vi "Create False Constant.vi"(5 "Sink":refnum<vi>, 6 "relative position/next to refnum":T1, 8 "error in (no error)":errorcluster, 11 "Diagram":refnum<vi>) -> (0 "error out":errorcluster, 2 "Output Terminal":refnum<vi>, 3 "Constant ref":refnum<vi>)   [LabVIEW 2012, in "Scripting Tools.lvlib"]
uses:
  Scripting Tools.lvlib
  <vilib>/Utility/miscctls.llb/LVPointTypeDef.ctl
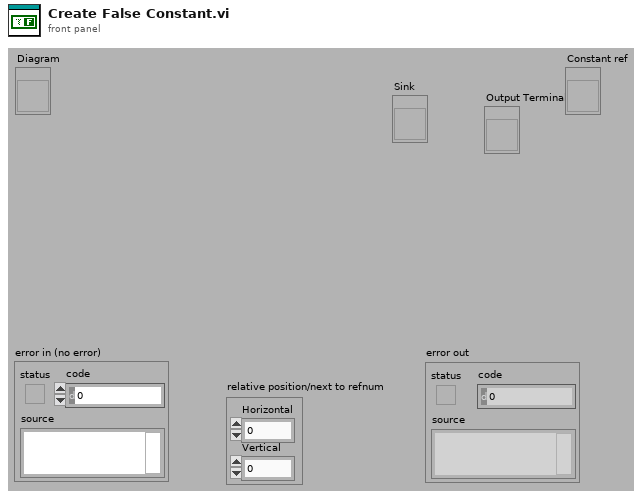
[diagram p1: front panel]
types:
  T1 = typedef "LVPointTypeDef.ctl" = cluster{"Horizontal":i16, "Vertical":i16}
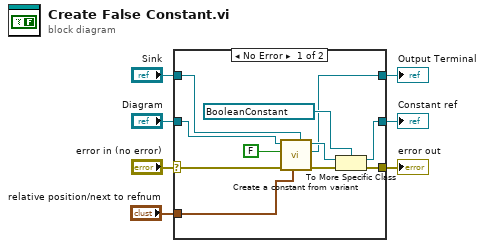
[diagram p0: block diagram]
diagram:
  n1 = case shown="No Error" "error in (no error)" {
    selector: "error in (no error)" -> [w16 w19]
    tunnel: "Diagram" -> [w18 _]
    tunnel: [w10 w19] -> w7
    tunnel: "relative position/next to refnum" -> [w15 _]
    tunnel: "Sink" -> [w14 _]
    tunnel: [w11 _] -> w2
    tunnel: [w8 _] -> w1
    frame No Error {
      n2 = call <userlib>:"Create a constant from variant.vi"("Terminal Sink"=w14, "relative position/next to refnum"=w15, "error in (no error)"=w16, "Constant Data"=FALSE, "Diagram"=w18) -> ("error out"=w9:errorcluster, "Terminal"=w8:refnum<vi>, "Const Refnum"=w13:refnum<vi>)  [unwired: 4 out]
      n3 = To More Specific Class(target class=refnum<vi> refnum ("reference out"), reference=w13, error in=w9) -> (specific class reference=w11:refnum<vi>, error out=w10:errorcluster)
    }
    frame Error {
    }
  }
  "Output Terminal" <- w1
  "error out" <- w7
  "Constant ref" <- w2
